vi "VI Server_TREE_ChildRowHeaders_GET.vi"(8 "error in (no error)":errorcluster, 9 "TreeControl in":refnum<vi>, 10 "Parent.RowHeader":string="1") -> (0 "error out":errorcluster, 1 "TreeControl.DUP":refnum<vi>, 4 "ChildRowHeaders":string[](array[string]))   [LabVIEW 2020]
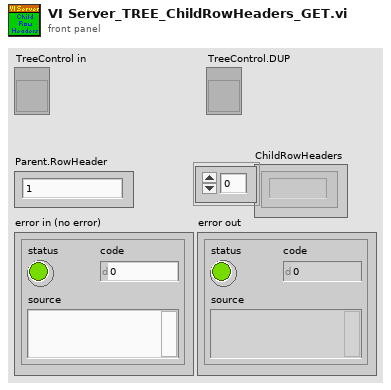
[diagram p1: front panel]
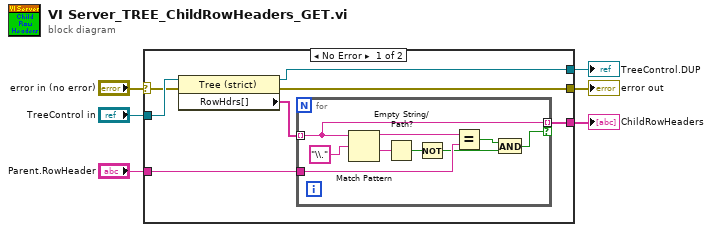
[diagram p0: block diagram]
diagram:
  n1 = case shown="No Error" "error in (no error)" {
    selector: "error in (no error)" -> [w9 w23]
    tunnel: "TreeControl in" -> [w13 _]
    tunnel: [w8 _] -> w3
    tunnel: "Parent.RowHeader" -> [w11 _]
    tunnel: [w10 w23] -> w5
    tunnel: [w7 _] -> w1
    frame No Error {
      n2 = property class="Tree (strict)"(reference=w13, error in=w9) -> (reference out=w7:refnum<vi>, error out=w10:errorcluster, "RowHdrs[]"=w12:string[])
      n3 = for {
        tunnel: w12 -> [w21] mode=indexing
        tunnel: [w21] -> w8 mode=indexing if=w14
        tunnel: w11 -> [w19]
        n4 = Match Pattern(string=w21, regular expression="\\.") -> (before substring=w20:string, after substring=w18:string)  [unwired: 1 in, 2 out]
        n5 = Empty String/Path?(string/path=w18) -> (empty?=w17:bool)
        n6 = Not(x=w17) -> (.not. x?=w16:bool)
        n7 = Equal?(x=w20, y=w19) -> (x = y?=w15:bool)
        n8 = And(x=w15, y=w16) -> (x .and. y?=w14:bool)
      }
    }
    frame Error {
    }
  }
  "ChildRowHeaders" <- w3
  "error out" <- w5
  "TreeControl.DUP" <- w1
